vi "test_launchTaskWithInvalidConnectorPaneShouldReturnError1031.vi"(11 "Test Case In":refnum<class "TaskControllerTests.lvclass">) -> (0 "error out":errorcluster, 3 "Test Case Out":refnum<class "TaskControllerTests.lvclass">)   [LabVIEW 2023, in "TaskControllerTests.lvclass"]
uses:
  TaskControllerTests.lvclass
  TaskMock/TaskMock.lvclass
  C:/projects/TLC_Daemon/source/ITask/ITask.lvclass
  TaskControllerTests.lvclass/TaskControllerTests.ctl
  source/TaskController/TaskController.lvclass
  <vilib>/Astemes/LUnit/Palette/Advanced Assertions/LUnit Advanced Assertions.lvlib
  C:/Program Files (x86)/National Instruments/LabVIEW 2023/vi.lib/Astemes/LUnit/Test Case.lvclass
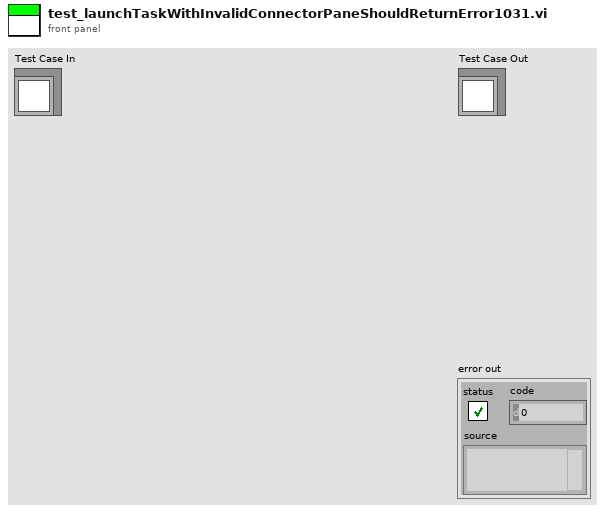
[diagram p1: front panel]
types:
  T1 = enum16{"ValidTask", "BrokenTask", "InvalidConnectorPaneTask"}
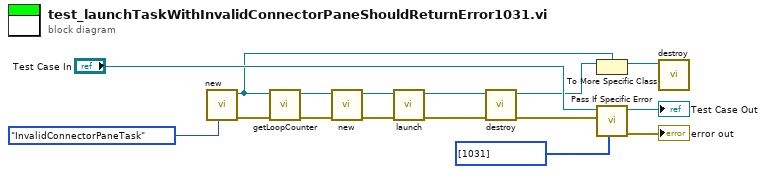
[diagram p0: block diagram]
diagram:
  n1 = call "new.vi"("taskType"=T1."InvalidConnectorPaneTask") -> ("error out"=w6:errorcluster, "TaskMock out"=w9:refnum<class "TaskMock.lvclass">)  [unwired: 9 in]
  n2 = call "getLoopCounter.vi"("error in (no error)"=w6, "TaskMock in"=w9) -> ("error out"=w5:errorcluster, "TaskMock out"=w11:refnum<class "TaskMock.lvclass">)  [unwired: 7 in, 1 out]
  n3 = call "new.vi"("error in (no error)"=w5, "task"=w11) -> ("error out"=w12:errorcluster, "TaskController out"=w13:refnum<class "TaskController.lvclass">)  [unwired: 8 in]
  n4 = call "launch.vi"("error in (no error)"=w12, "TaskController in"=w13) -> ("error out"=w3:errorcluster, "TaskController out"=w10:refnum<class "TaskController.lvclass">)  [unwired: 8 in]
  n5 = call "destroy.vi"("error in (no error)"=w3, "TaskController in"=w10) -> ("error out"=w1:errorcluster, "taskResult"=w8:refnum<class "ITask.lvclass">)  [unwired: 8 in]
  n6 = To More Specific Class(target class=w9, reference=w8) -> (specific class reference=w7:refnum<class "TaskMock.lvclass">)  [unwired: 1 in, 1 out]
  n7 = call <vilib>:"Pass If Specific Error.vi"("Error Codes"=i32[] [1031], "Assert error"=w1, "LUnit Test Case In"="Test Case In") -> ("error out"=→"error out":errorcluster, "LUnit Test Case Out"=→"Test Case Out":refnum<class "TaskControllerTests.lvclass">)  [unwired: 7 in]
  n8 = call "destroy.vi"("TaskMock in"=w7) -> ()  [unwired: 10 in, 1 out]
